vi "Menu Search By Tag Array.vi"(8 "error in (no error)":errorcluster, 10 "Tag Array":string[](array[string]), 11 "Menu MGI Ref":refnum<class "MGI_VI.lvclass">) -> (0 "error out":errorcluster, 2 "Found?":bool[](array[boolean]), 3 "Menu Item Array":refnum<data-value>[](array[refnum]))   [LabVIEW 2018, in "LF2R IDE.lvlib" / "LF2R IDE.lvclass"]
uses:
  LF2R IDE.lvclass
  <userlib>/_MGI/Menu Building/MenuTypes/Vi/MGI_VI.lvclass
  C:/Program Files (x86)/National Instruments/LabVIEW 2018/user.lib/_MGI/Menu Building/MenuTypes/MGI_Menu.lvclass
  <userlib>/_MGI/Menu Building/MenuItem/MGI_MenuItem.lvclass
  <userlib>/_MGI/Menu Building/MenuTypes/Read Menu Items.vi
  <userlib>/_MGI/Menu Building/MenuItem/Read Sub-Menus.vi
  <userlib>/_MGI/Menu Building/MenuItem/Read Tag.vi
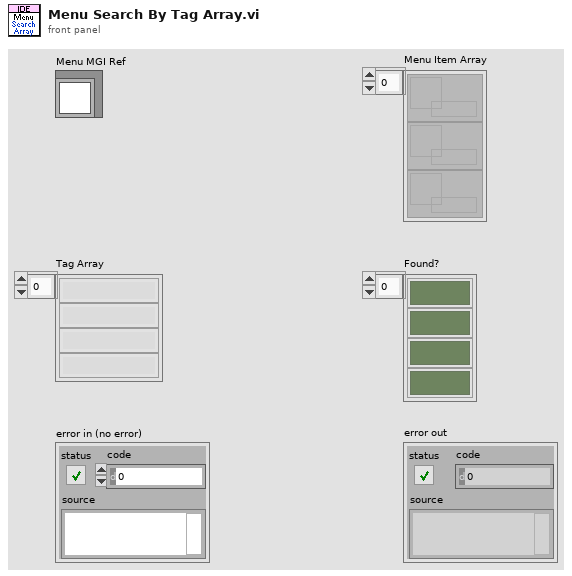
[diagram p1: front panel]
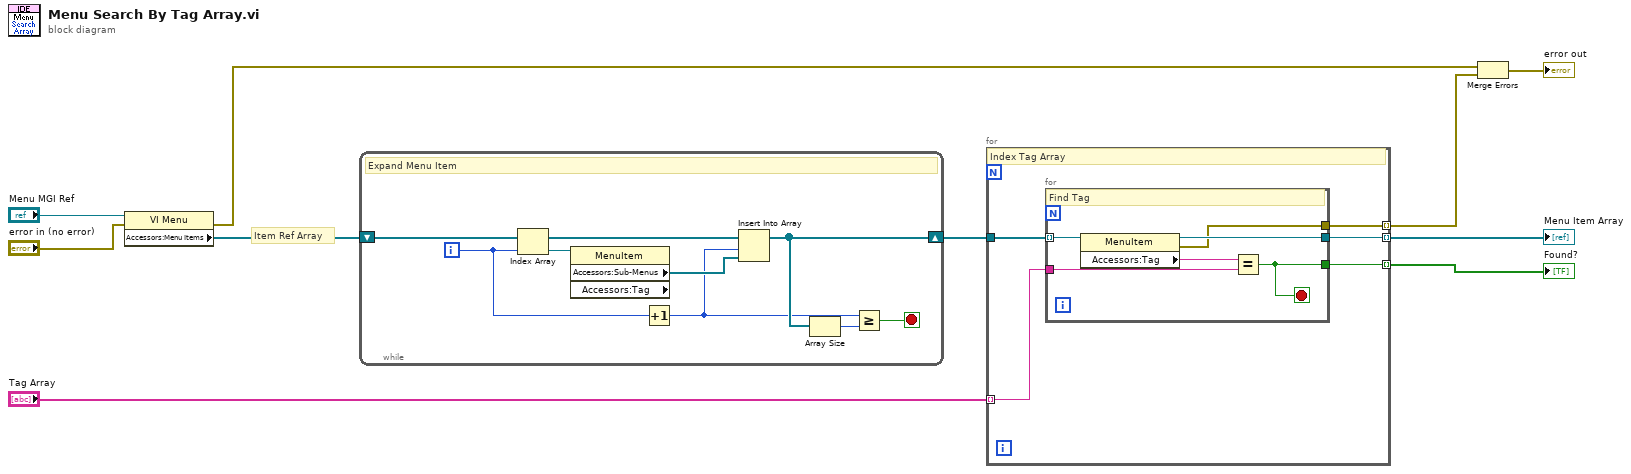
[diagram p0: block diagram]
diagram:
  # "Item Ref Array"
  n1 = property class="VI Menu"(reference="Menu MGI Ref", error in="error in (no error)") -> (error out=w5:errorcluster, "Accessors:Menu Items"=w10:refnum<data-value>[])  [unwired: 1 out]
  n2 = while {
    shift-right: [w14] -> w8
    shift-left: w10 -> [w17]
    i -> [w15]
    stop <- w11 stop-if-true
    # "Expand Menu Item"
    n3 = Index Array(array=w17, index=w15) -> (element=w18:refnum<data-value>)
    n4 = property class="MenuItem" props=["Accessors:Sub-Menus", "Accessors:Tag"](reference=w18) -> ("Accessors:Sub-Menus"=w16:refnum<data-value>[])  [unwired: 1 in, 3 out]
    n5 = Increment(x=w15) -> (x+1=w12:i32)
    n6 = Insert Into Array(array=w17, index=w12, new element=w16) -> (w14:refnum<data-value>[])
    n7 = Array Size(array=w14) -> (size(s)=w13:i32)
    n8 = Greater Or Equal?(x=w12, y=w13) -> (x >= y?=w11:bool)
  }
  n9 = for {
    tunnel: w8 -> [w23]
    tunnel: [w22] -> w2 mode=indexing
    tunnel: [w21] -> w6 mode=indexing
    tunnel: "Tag Array" -> [w20] mode=indexing
    tunnel: [w19] -> w1 mode=indexing
    # "Index Tag Array"
    n10 = for {
      tunnel: [w24] -> w19
      tunnel: [w26] -> w21
      tunnel: w20 -> [w25]
      tunnel: w23 -> [w29] mode=indexing
      tunnel: [w27] -> w22
      stop <- w24 stop-if-true
      # "Find Tag"
      n11 = property class="MenuItem"(reference=w29) -> (reference out=w27:refnum<data-value>, error out=w26:errorcluster, "Accessors:Tag"=w28:string)  [unwired: 1 in]
      n12 = Equal?(x=w28, y=w25) -> (x = y?=w24:bool)
    }
  }
  "Menu Item Array" <- w2
  "Found?" <- w1
  n13 = Merge Errors(w5, w6) -> (→"error out":errorcluster)
